vi "createSubDataEvents.vi"(8 "error in (no error)":errorcluster, 11 "UserEvents in":refnum<class "UserEvents.lvclass">) -> (0 "error out":errorcluster, 3 "UserEvents out":refnum<class "UserEvents.lvclass">)   [LabVIEW 2012, in "UserEvents.lvclass"]
uses:
  UserEvents.lvclass
  UserEvents.lvclass/UserEvents.ctl
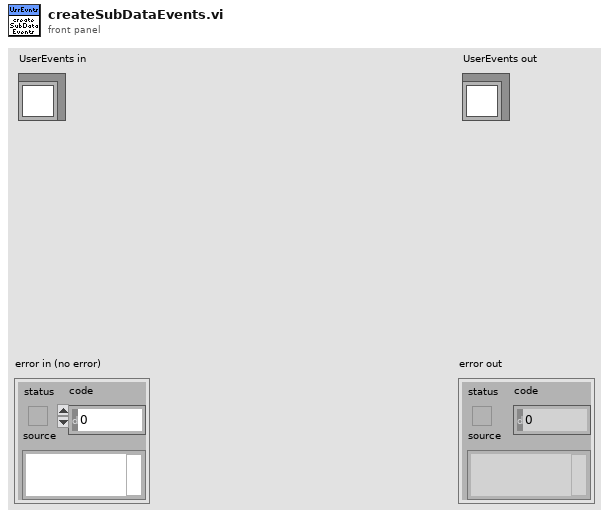
[diagram p1: front panel]
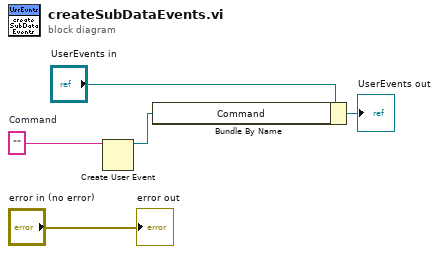
[diagram p0: block diagram]
diagram:
  w2 = ""  # Command
  n1 = Create User Event(user event datatype=w2) -> (user event=w1:refnum<user-event>)  [unwired: 1 in, 1 out]
  n2 = Bundle By Name(cluster="UserEvents in", "Command"=w1) -> (→"UserEvents out":refnum<class "UserEvents.lvclass">)
  "error out" <- "error in (no error)"
